vi "svx_Probe Angle Preprocess.vi"(8 "channel name Y":string, 9 "channel name X":string, 10 "Y":u16, 11 "X":u16) -> (0 "actual Y":string, 1 "actual X":string, 2 "Y":dbl, 3 "X":dbl, 5 "switched?":bool)   [LabVIEW 2017]
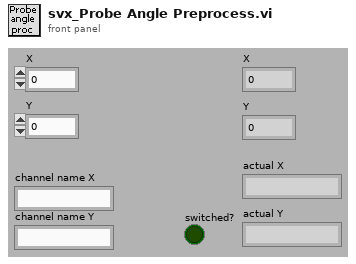
[diagram p1: front panel]
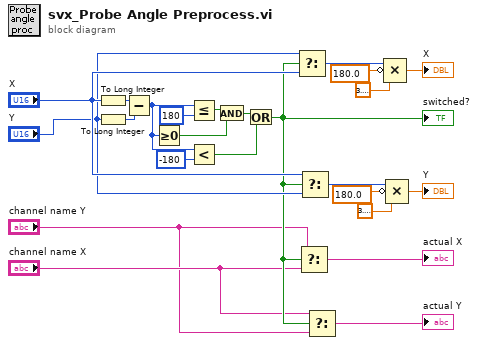
[diagram p0: block diagram]
diagram:
  n1 = To Long Integer(number="X") -> (32bit integer=w16:i32)
  n2 = To Long Integer(number="Y") -> (32bit integer=w24:i32)
  n3 = Subtract(x=w16, y=w24) -> (x-y=w20:i32)
  n4 = Greater Or Equal To 0?(x=w20) -> (x >= 0?=w21:bool)
  n5 = Less Or Equal?(x=w20, y=u32 180) -> (x <= y?=w22:bool)
  n6 = Less?(x=w20, y=-180) -> (x < y?=w17:bool)
  n7 = And(x=w22, y=w21) -> (x .and. y?=w18:bool)
  n8 = Or(x=w18, y=w17) -> (x .or. y?=w5:bool)
  "switched?" <- w5
  n9 = Select(t="Y", s=w5, f="X") -> (s? t:f=w13:u16)
  n10 = Select(t="channel name Y", s=w5, f="channel name X") -> (s? t:f=→"actual X":string)
  n11 = Select(t="X", s=w5, f="Y") -> (s? t:f=w10:u16)
  n12 = Select(t="channel name X", s=w5, f="channel name Y") -> (s? t:f=→"actual Y":string)
  n13 = Compound Arithmetic op=MULTIPLY(w13, invert 180.0 ("value"), 3.141592653589793) -> (→"X":dbl)
  n14 = Compound Arithmetic op=MULTIPLY(w10, invert 180.0 ("value"), 3.141592653589793) -> (→"Y":dbl)
